vi "SMSD_position_format.vi"(11 "DATA":u8[](array[numeric])) -> (3 "position":i32)   [LabVIEW 2019, in "SMSD.lvclass"]
uses:
  SMSD.lvclass
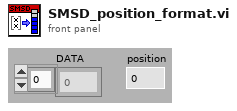
[diagram p1: front panel]
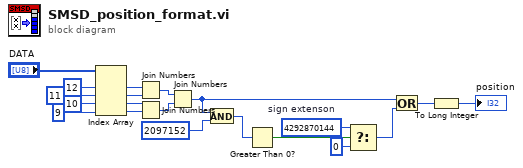
[diagram p0: block diagram]
diagram:
  w7 = u32 4292870144  # sign extenson
  n1 = Index Array(array="DATA", index #1=12 ("index"), index #2=11 ("index"), index #3=10 ("index"), index #4=9 ("index")) -> (element #1=w17:u8, element #2=w16:u8, element #3=w15:u8, element #4=w14:u8)
  n2 = Join Numbers(hi=w17, lo=w16) -> ((hi.lo)=w13:u16)
  n3 = Join Numbers(hi=w15, lo=w14) -> ((hi.lo)=w12:u16)
  n4 = Join Numbers(hi=w13, lo=w12) -> ((hi.lo)=w5:u32)
  n5 = And(x=w5, y=u32 2097152) -> (x .and. y?=w9:u32)
  n6 = Greater Than 0?(x=w9) -> (x > 0?=w8:bool)
  n7 = Select(t=w7, s=w8, f=u32 0) -> (s? t:f=w4:u32)
  n8 = Or(x=w5, y=w4) -> (x .or. y?=w2:u32)
  n9 = To Long Integer(number=w2) -> (32bit integer=→"position":i32)
